vi "Material-WidenCalPulses.vi"(0 "raw CAL indexes":u32[](array[numeric])=[308, 309, 310, 311, 312, 313, 314, 315, 316, 317, 318, 319, 320, 321, 322, 323, 324, 325, 326, 327, 328, 329, 330, 331, 1444, 1445, 1446, 1447, 1448, 1449, 1450, 1451, 1452, 1453, 1454, 1455, 1456, 1457, 1458, 1459, 1460, 1461, 1462, 1463, 1464, 1465, 1466, 1467, 1468, 2009]) -> (1 "New Indexes":u32[](array[numeric]))   [LabVIEW 2013, in "Material-RunTest.lvclass"]
uses:
  Material-RunTest.lvclass
panel:
  out "element":i32
  out "array w/ subset deleted":u32[][](array[numeric])
  out "Array 2":u32[][](array[numeric])
  out "Extended Cal indexes":u32[](array[numeric])
  out "subarray":u32[](array[numeric])
  out "max value":u32
  out "Array":u32[](array[numeric])
  out "x = y?":bool
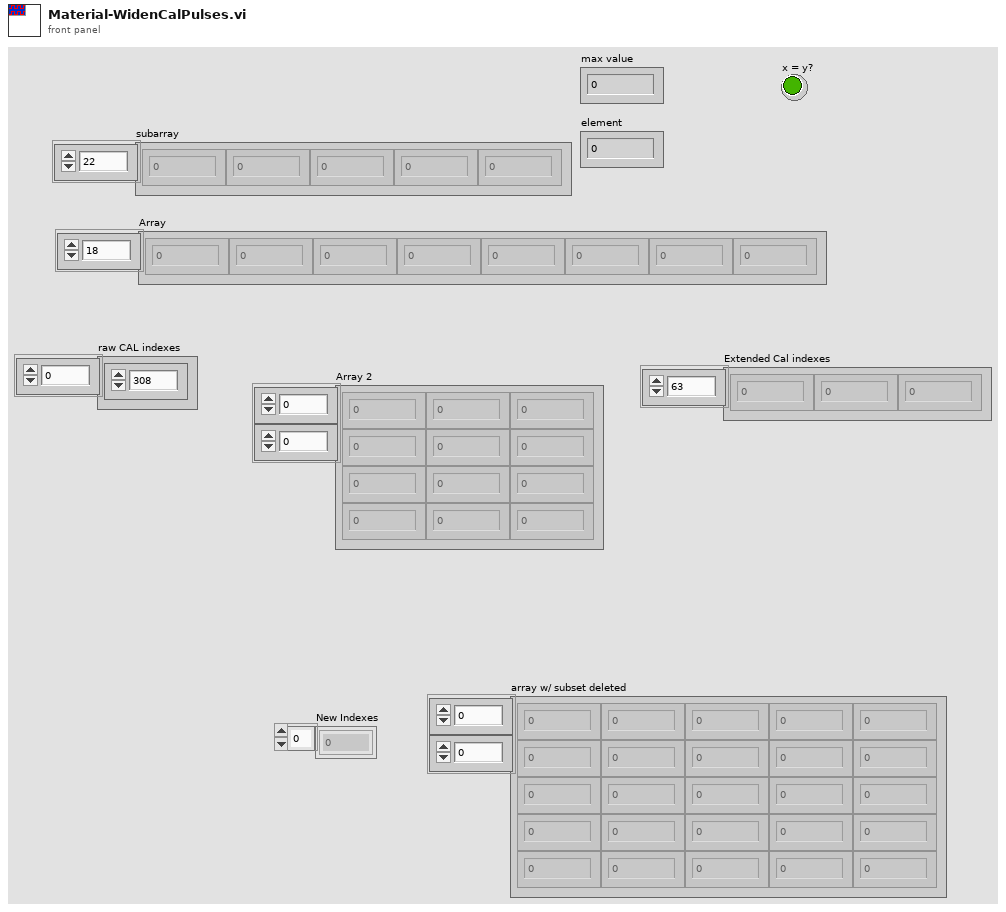
[diagram p1: front panel]
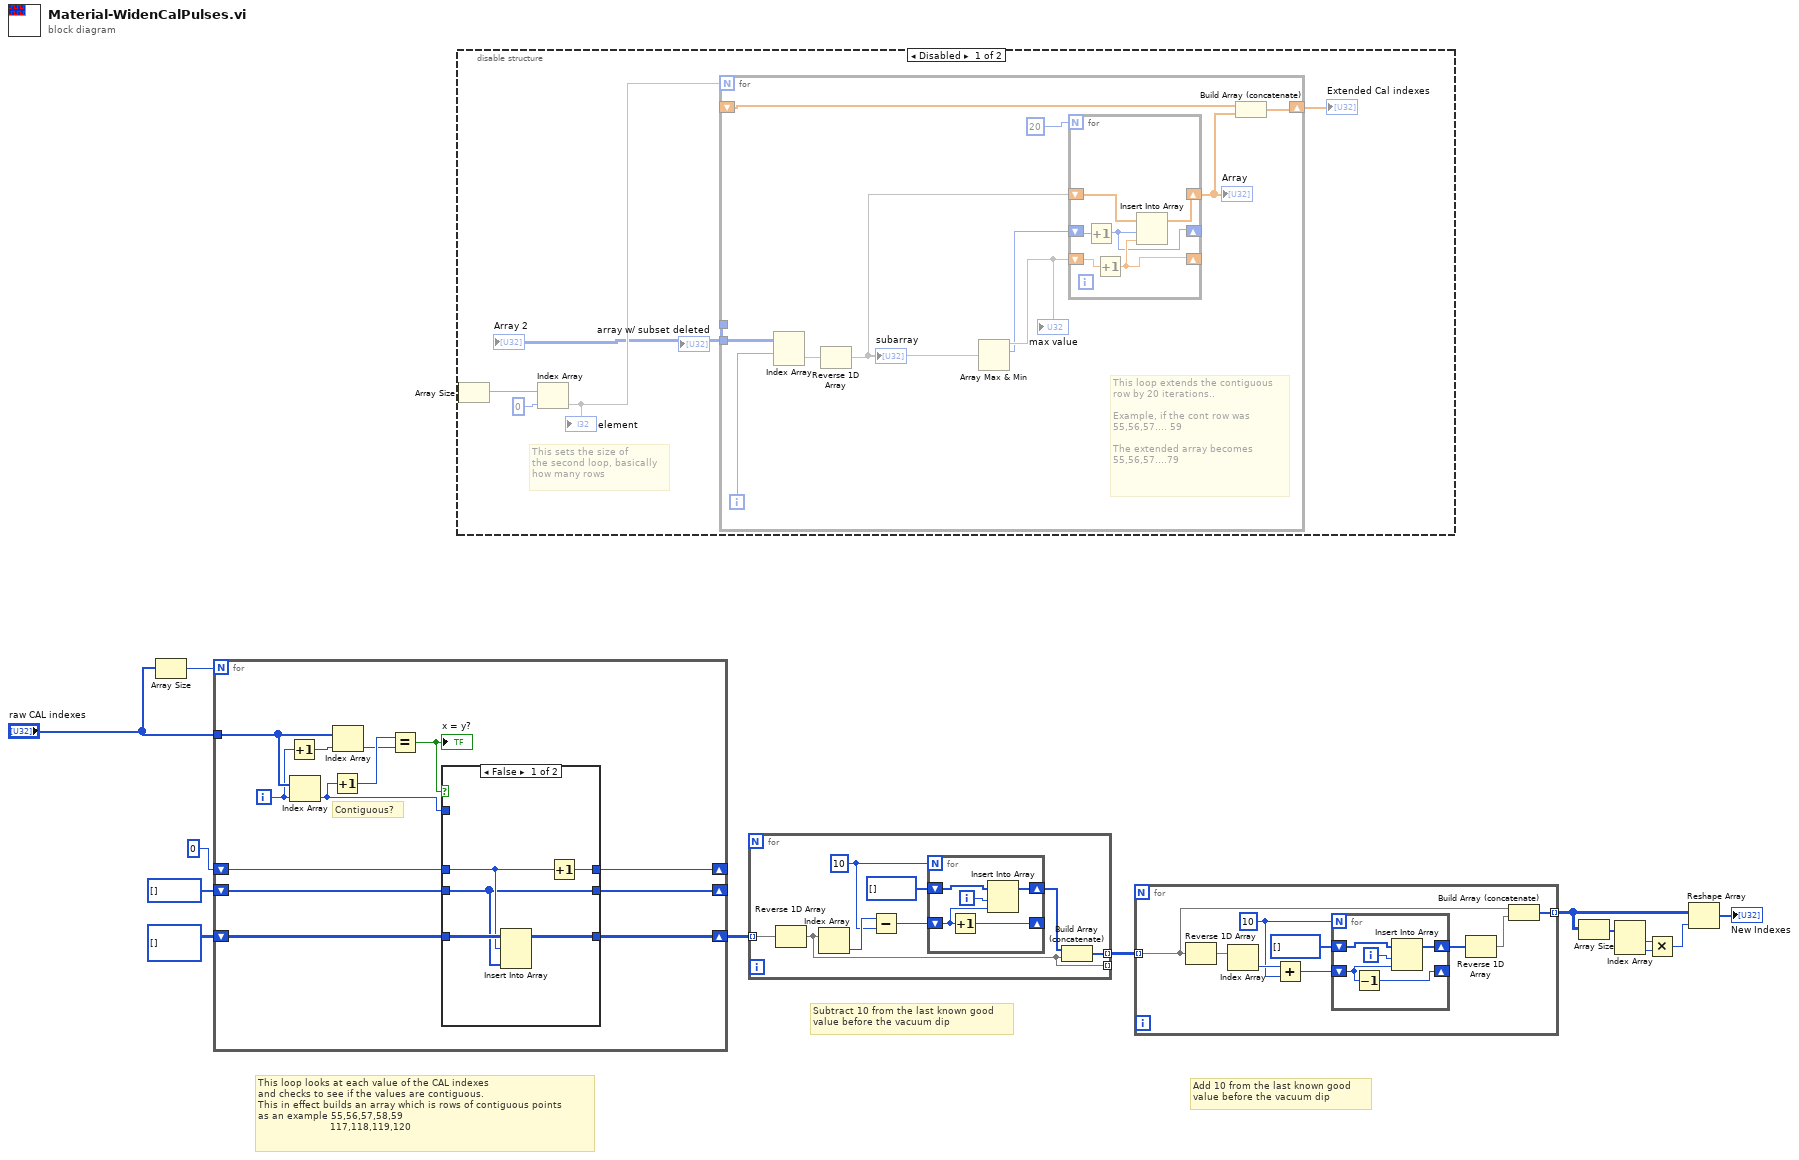
[diagram p0: block diagram]
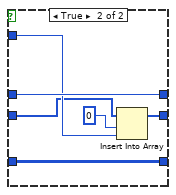
[diagram p3: hidden frame]
diagram:
  # "Add 10 from the last known good\nvalue before the vacuum dip"
  # "Subtract 10 from the last known good\nvalue before the vacuum dip"
  # "This loop looks at each value of the CAL indexes\nand checks to see if the values are contiguous.\nThis in effect builds an array which is rows of contiguous points\nas an example 55,56,57,58,59\n                        117,118,119,120"
  n1 = Array Size(array="raw CAL indexes") -> (size(s)=w12:i32)
  n2 = for {
    N: w12 -> [_]
    tunnel: "raw CAL indexes" -> [w26]
    shift-right: [w14] -> _
    shift-left: u32[] [] -> [w17]
    shift-right: [w20] -> _
    shift-left: 0 ("x+1 2") -> [w21]
    shift-right: [w15] -> w7
    shift-left: u32[][] [] ("Array") -> [w16]
    i -> [w24]
    # "Contiguous?"
    n3 = Increment(x=w24) -> (x+1=w25:i32)
    n4 = Index Array(array=w26, index=w24) -> (element=w18:u32)
    n5 = Increment(x=w18) -> (x+1=w23:u32)
    n6 = Index Array(array=w26, index=w25) -> (element=w22:u32)
    n7 = Equal?(x=w23, y=w22) -> (x = y?=w19:bool)
    "x = y?" <- w19
    n8 = case shown="False" w19 {
      tunnel: [w31 w37] -> w20
      tunnel: w21 -> [w28 w37]
      tunnel: w18 -> [_ w36]
      tunnel: [w27 w33] -> w14
      tunnel: w17 -> [w27 w35]
      tunnel: w16 -> [w30 w32]
      tunnel: [w29 w32] -> w15
      frame False {
        n9 = Insert Into Array(array=w30, index (row)=w28, new element=w27) -> (w29:u32[][])  [unwired: 1 in]
        n10 = Increment(x=w28) -> (x+1=w31:i32)
      }
      frame True {
        n11 = Insert Into Array(array=w35, index=0, new element=w36) -> (w33:u32[])
      }
    }
  }
  n12 = disable-structure shown="Disabled" {
    frame Disabled {
      # "This sets the size of\nthe second loop, basically\nhow many rows"
      n13 = Array Size() -> (size(s)=w42:i32)  [unwired: 1 in]
      n14 = Index Array(array=w42, index=0) -> (element=w39)
      "element" <- w39
      n15 = for {
        N: w39 -> [_]
        tunnel: [w44] -> _
        shift-right: [w45] -> w40
        shift-left: _ -> [w46]
        tunnel: "Array 2" -> [w44]
        i -> [w48]
        # "This loop extends the contiguous\nrow by 20 iterations..\n\nExample, if the cont row was\n55,56,57.... 59\n\nThe extended array becomes\n55,56,57....79"
        n16 = Index Array(array=w44, index (row)=w48) -> (element=w43)  [unwired: 1 in]
        n17 = Reverse 1D Array(array=w43) -> (reversed array=w51:void[])
        "subarray" <- w51
        n18 = Array Max & Min(array=w51) -> (max value=w50, max index (indices)=w49:i32)  [unwired: 2 out]
        "max value" <- w50
        n19 = for {
          N: 20 -> [_]
          shift-right: [w58] -> w47
          shift-left: w51 -> [w57]
          shift-right: [w55] -> _
          shift-left: w50 -> [w56]
          shift-right: [w53] -> _
          shift-left: w49 -> [w54]
          n20 = Increment(x=w54) -> (x+1=w53:i32)
          n21 = Increment(x=w56) -> (x+1=w55:dbl)
          n22 = Insert Into Array(array=w57, index=w53, new element=w55) -> (w58:dbl[])
        }
        "Array" <- w47
        n23 = Build Array (concatenate)(w46, w47) -> (w45:dbl[])
      }
      "Extended Cal indexes" <- w40
    }
    frame Enabled {
    }
  }
  n24 = for {
    tunnel: w7 -> [w61] mode=indexing
    tunnel: [w62] -> w8 mode=indexing
    tunnel: [w59] -> _ mode=indexing
    w64 = u32 10 ("y")
    n25 = Reverse 1D Array(array=w61) -> (reversed array=w59:u32[])
    n26 = Index Array(array=w59) -> (element=w66:u32)  [unwired: 1 in]
    n27 = Subtract(x=w66, y=w64) -> (x-y=w65:u32)
    n28 = for {
      N: w64 -> [_]
      shift-right: [w70] -> w60
      shift-left: i32[] [] -> [w71]
      shift-right: [w67] -> _
      shift-left: w65 -> [w68]
      i -> [w69]
      n29 = Increment(x=w68) -> (x+1=w67:u32)
      n30 = Insert Into Array(array=w71, index=w69, new element=w68) -> (w70:i32[])
    }
    n31 = Build Array (concatenate)(w60, w59) -> (w62:u32[])
  }
  n32 = for {
    tunnel: w8 -> [w76] mode=indexing
    tunnel: [w75] -> w2 mode=indexing
    w74 = u32 10 ("y")
    n33 = Reverse 1D Array(array=w76) -> (reversed array=w79:u32[])
    n34 = Index Array(array=w79) -> (element=w80:u32)  [unwired: 1 in]
    n35 = Add(x=w80, y=w74) -> (x+y=w77:u32)
    n36 = for {
      N: w74 -> [_]
      shift-right: [w84] -> w73
      shift-left: i32[] [] -> [w85]
      shift-right: [w81] -> _
      shift-left: w77 -> [w82]
      i -> [w83]
      n37 = Decrement(x=w82) -> (x-1=w81:u32)
      n38 = Insert Into Array(array=w85, index=w83, new element=w82) -> (w84:i32[])
    }
    n39 = Reverse 1D Array(array=w73) -> (reversed array=w72:i32[])
    n40 = Build Array (concatenate)(w76, w72) -> (w75:u32[])
  }
  n41 = Array Size(array=w2) -> (size(s)=w6:i32[])
  n42 = Index Array(array=w6) -> (element #1=w5:i32, element #2=w4:i32)  [unwired: 2 in]
  n43 = Multiply(x=w5, y=w4) -> (x*y=w3:i32)
  n44 = Reshape Array(w2, w3) -> (→"New Indexes":u32[])
